vi "ToggleSolenoidOnPressForDoubleAction 2.vi"(11 "Button":bool) -> (3 "Value":T1)   [LabVIEW 2018]
uses:
  <vilib>/Rock Robotics/WPI/Solenoid/WPI_SolenoidValue.ctl
panel:
  # "Create a Toggle Action Solenoid on a \nSingle Button Press"
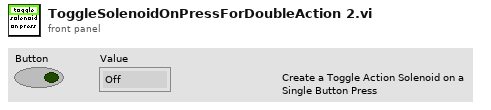
[diagram p1: front panel]
types:
  T1 = typedef "WPI_SolenoidValue.ctl" = enum16{"Off", "On", "Forward", "Reverse"}
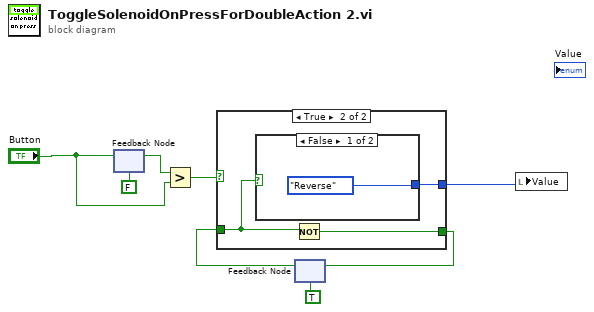
[diagram p0: block diagram]
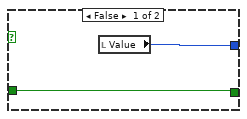
[diagram p2: hidden frame]
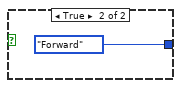
[diagram p3: hidden frame]
diagram:
  n1 = feedback #1(FALSE) -> (w4:bool)
  n2 = feedback-in #1("Button") -> ()
  n3 = Greater?(x=w4, y="Button") -> (0:w6:bool)
  n4 = feedback #2(TRUE) -> (w7:bool)
  n5 = case shown="True" w6 {
    tunnel: w7 -> [w10 w13]
    tunnel: [w10 w12] -> w8
    tunnel: [w9 w11] -> w2
    frame False {
      n6 = local read "Value"() -> (w9:T1)
    }
    frame True {
      n7 = case shown="False" w13 {
        tunnel: [WPI_SolenoidValue."Reverse" ("Value") WPI_SolenoidValue."Forward" ("Value")] -> w11
        frame False {
        }
        frame True {
        }
      }
      n8 = Not(x=w13) -> (.not. x?=w12:bool)
    }
  }
  n9 = feedback-in #2(w8) -> ()
  n10 = local write "Value"(w2) -> ()
